vi "STL-ArrayToCanvas.vi"(9 "Scale":i32=50, 10 "STL array":dbl[][](array[numeric]), 11 "Picture In":picture) -> (3 "Picture Out":picture)   [LabVIEW 2019]
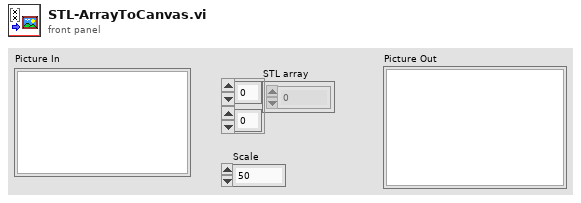
[diagram p1: front panel]
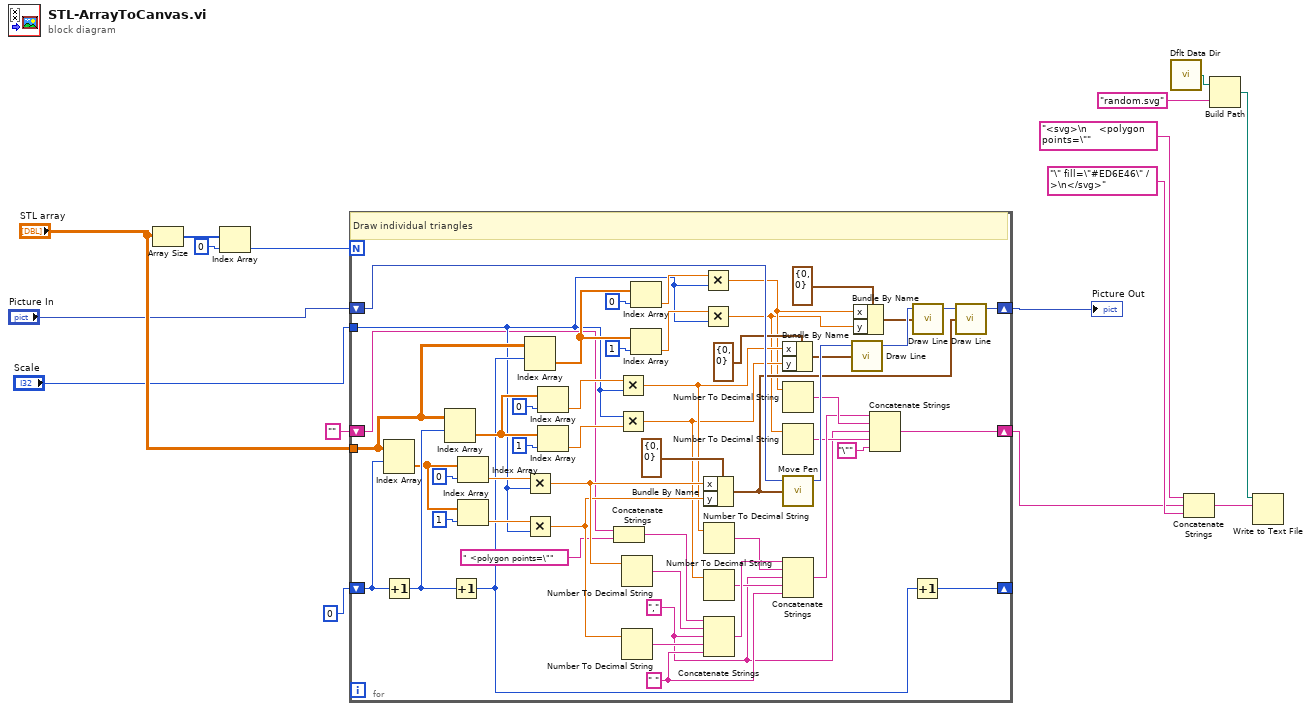
[diagram p0: block diagram]
diagram:
  n1 = Array Size(array="STL array") -> (size(s)=w14:i32[])
  n2 = Index Array(array=w14, index=0) -> (element=w16:i32)
  n3 = for {
    N: w16 -> [_]
    tunnel: "STL array" -> [w68]
    shift-right: [w41] -> _
    shift-left: 0 -> [w44]
    shift-right: [w39] -> w11
    shift-left: "Picture In" -> [w67]
    tunnel: "Scale" -> [w45]
    shift-right: [w37] -> w2
    shift-left: "" -> [w20]
    w27 = " " ("string")
    w17 = "," ("string")
    # "Draw individual triangles"
    n4 = Index Array(array=w68, index (row)=w44) -> (element=w58:dbl[])  [unwired: 1 in]
    n5 = Increment(x=w44) -> (x+1=w69:i32)
    n6 = Index Array(array=w68, index (row)=w69) -> (element=w57:dbl[])  [unwired: 1 in]
    n7 = Increment(x=w69) -> (x+1=w46:i32)
    n8 = Index Array(array=w58, index=0) -> (element=w52:dbl)
    n9 = Index Array(array=w58, index=1) -> (element=w51:dbl)
    n10 = Index Array(array=w68, index (row)=w46) -> (element=w56:dbl[])  [unwired: 1 in]
    n11 = Multiply(x=w52, y=w45) -> (x*y=w36:dbl)
    n12 = Multiply(x=w51, y=w45) -> (x*y=w34:dbl)
    n13 = Index Array(array=w57, index=0) -> (element=w50:dbl)
    n14 = Index Array(array=w57, index=1) -> (element=w49:dbl)
    n15 = Concatenate Strings(w20, " <polygon points=\"" ("string")) -> (w18:string)
    n16 = Multiply(x=w50, y=w45) -> (x*y=w31:dbl)
    n17 = Multiply(x=w45, y=w49) -> (x*y=w29:dbl)
    n18 = Number To Decimal String(number=w36) -> (decimal integer string=w35:string)  [unwired: 1 in]
    n19 = Number To Decimal String(number=w34) -> (decimal integer string=w33:string)  [unwired: 1 in]
    n20 = Index Array(array=w56, index=0) -> (element=w48:dbl)
    n21 = Index Array(array=w56, index=1) -> (element=w47:dbl)
    n22 = Multiply(x=w48, y=w45) -> (x*y=w26:dbl)
    n23 = Multiply(x=w47, y=w45) -> (x*y=w22:dbl)
    n24 = Bundle By Name(cluster=cluster{"x":i16, "y":i16} {"x"=0, "y"=0} ("end point"), "x"=w36, "y"=w34) -> (w38:cluster{"x":i16, "y":i16})
    n25 = Number To Decimal String(number=w31) -> (decimal integer string=w30:string)  [unwired: 1 in]
    n26 = Number To Decimal String(number=w29) -> (decimal integer string=w28:string)  [unwired: 1 in]
    n27 = Concatenate Strings(w18, w35, w17, w33, w27) -> (w32:string)
    n28 = Bundle By Name(cluster=cluster{"x":i16, "y":i16} {"x"=0, "y"=0} ("end point"), "x"=w31, "y"=w29) -> (w42:cluster{"x":i16, "y":i16})
    n29 = Number To Decimal String(number=w26) -> (decimal integer string=w25:string)  [unwired: 1 in]
    n30 = Number To Decimal String(number=w22) -> (decimal integer string=w23:string)  [unwired: 1 in]
    n31 = call <vilib>:"Move Pen.vi"("new position"=w38, "picture"=w67) -> ("new picture"=w66:picture)  [unwired: 3 in]
    n32 = Concatenate Strings(w32, w30, w17, w28, w27) -> (w24:string)
    n33 = call <vilib>:"Draw Line.vi"("picture"=w66, "end point"=w42) -> ("new picture"=w65:picture)  [unwired: 7 in]
    n34 = Bundle By Name(cluster=cluster{"x":i16, "y":i16} {"x"=0, "y"=0} ("end point"), "x"=w26, "y"=w22) -> (w43:cluster{"x":i16, "y":i16})
    n35 = Concatenate Strings(w24, w25, w17, w23, "\"" ("string")) -> (w37:string)
    n36 = Increment(x=w46) -> (x+1=w41:i32)
    n37 = call <vilib>:"Draw Line.vi"("picture"=w65, "end point"=w43) -> ("new picture"=w40:picture)  [unwired: 7 in]
    n38 = call <vilib>:"Draw Line.vi"("picture"=w40, "end point"=w38) -> ("new picture"=w39:picture)  [unwired: 7 in]
  }
  "Picture Out" <- w11
  n39 = call <vilib>:"Dflt Data Dir.vi"() -> ("App:Default Data Directory"=w8:path)
  n40 = Concatenate Strings("<svg>\n    <polygon points=\"" ("string"), w2, "\" fill=\"#ED6E46\" />\n</svg>") -> (w3:string)
  n41 = Build Path(base path=w8, name or relative path="random.svg") -> (appended path=w6:path)
  n42 = Write to Text File(file (use dialog)=w6, text=w3) -> ()  [unwired: 2 in, 3 out]
